vi "Update Data.vi"(8 "error in (no error)":errorcluster, 9 "data":waveform(dbl)[](array[waveform]), 10 "Channel Names":string[](array[string]), 11 "Data Interface in":refnum<class "Data Interface.lvclass">) -> (0 "error out":errorcluster, 3 "Data Interface out":refnum<class "Data Interface.lvclass">)   [LabVIEW 2020, in "Data Interface.lvclass"]
uses:
  Data Interface.lvclass
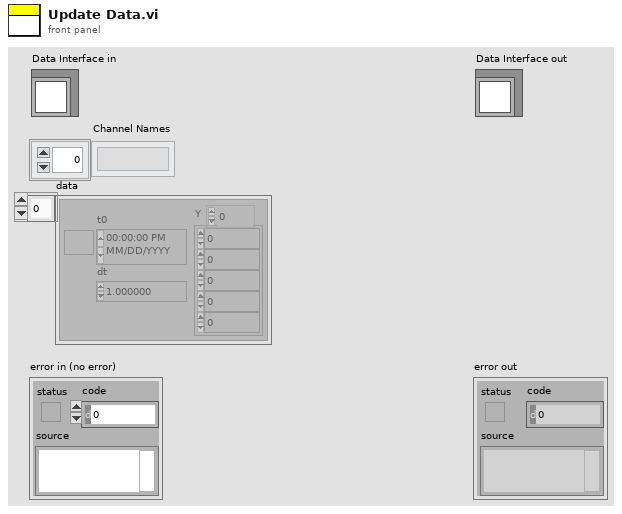
[diagram p1: front panel]
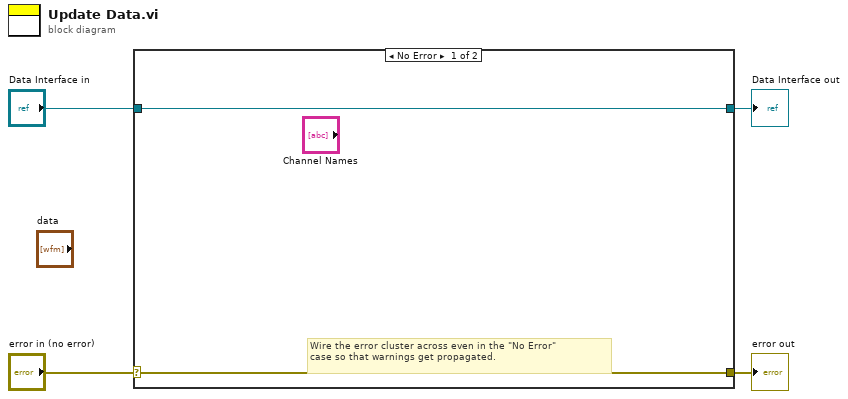
[diagram p0: block diagram]
diagram:
  n1 = case shown="No Error" "error in (no error)" {
    selector: "error in (no error)" -> [w5 w8]
    tunnel: [w5 w8] -> w3
    tunnel: [w6 w7] -> w1
    tunnel: "Data Interface in" -> [w6 w7]
    frame No Error {
      # "Wire the error cluster across even in the \"No Error\"\ncase so that warnings get propagated."
    }
    frame Error {
    }
  }
  "error out" <- w3
  "Data Interface out" <- w1
